vi "set_fiberdrive_parameters.vi"(8 "error in (no error)":errorcluster, 10 "Fiber spiral parameters":T1={"Fiber Frequency"=2200, "Imaging Periods"=100, "Settling Periods"=50, "Resting Periods"=30, "Amplitude X"=0.5, "Amplitude Y"=0.5, "Phase difference"=90.0, "Initial Amplitude X"=0.0, "Initial Amplitude Y"=0.0} {"Initial Amplitude Y" min=0.0 max=3.0 step=0.1; "Initial Amplitude X" min=0.0 max=3.0 step=0.1; "Phase difference" min=0.0 max=360.0 step=5.0; "Amplitude Y" min=0.0 max=3.0 step=0.1; "Amplitude X" min=0.0 max=3.0 step=0.1}, 11 "TrajectoryRK110428Fiber in":refnum<class "TrajectoryRK110428Fiber_Spiral.lvclass">) -> (0 "error out":errorcluster, 3 "TrajectoryRK110428Fiber out":refnum<class "TrajectoryRK110428Fiber_Spiral.lvclass">)   [LabVIEW 2010, in "TrajectoryRK110428Fiber_Spiral.lvclass"]
uses:
  TrajectoryRK110428Fiber_Spiral.lvclass
  FPGAWrapper/FPGAWrapperRK110512Fiber/FPGAWrapperRK110512Fiber_Spiral/fiber_spiral_parameters.ctl
  TrajectoryRK110428Fiber_Spiral.lvclass/TrajectoryRK110428Fiber_Spiral.ctl
  FPGAWrapper/FPGAWrapperRK110512Fiber/FPGAWrapperRK110512Fiber_Spiral/FPGAWrapperRK110512Fiber_Spiral.lvclass
panel:
  # "[Hz]"
  # "[V]"
  # "[V]"
  # "[deg]"
  # "[V]"
  # "[V]"
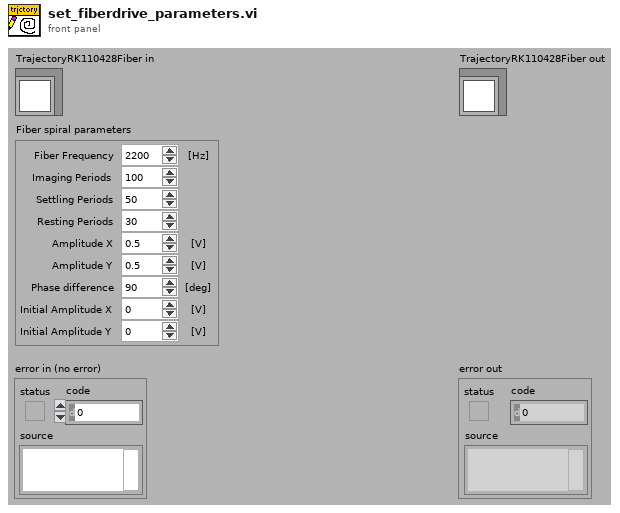
[diagram p1: front panel]
types:
  T1 = typedef "FPGAWrapperRK110512Fiber_Spiral.lvclass/fiber_spiral_parameters.ctl" = cluster{"Fiber Frequency":u16, "Imaging Periods":u16, "Settling Periods":u16, "Resting Periods":u16, "Amplitude X":dbl, "Amplitude Y":dbl, "Phase difference":dbl, "Initial Amplitude X":dbl, "Initial Amplitude Y":dbl}
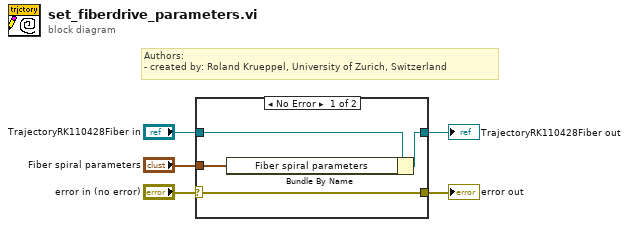
[diagram p0: block diagram]
diagram:
  # "Authors: \n- created by: Roland Krueppel, University of Zurich, Switzerland"
  n1 = case shown="No Error" "error in (no error)" {
    selector: "error in (no error)" -> [w9 w10]
    tunnel: [w9 w10] -> w4
    tunnel: [w7 w11] -> w2
    tunnel: "TrajectoryRK110428Fiber in" -> [w8 w11]
    tunnel: "Fiber spiral parameters" -> [w6 _]
    frame No Error {
      n2 = Bundle By Name(cluster=w8, "Fiber spiral parameters"=w6) -> (w7:refnum<class "TrajectoryRK110428Fiber_Spiral.lvclass">)
    }
    frame Error {
    }
  }
  "error out" <- w4
  "TrajectoryRK110428Fiber out" <- w2
